vi "Procesare.vi"() -> ()   [LabVIEW 2024]
uses:
  <vilib>/vision/NI_Vision_Development_Module.lvlib
panel:
  out "Image":T1(plugin-control)
  out "Image 1D array":dbl[](array[numeric])
  out "Inputs":i32
  out "Dimensiune Imagine":i32[](array[numeric])
  out "Array":dbl[][](array[numeric])
  in  "Productivitate  minima":dbl
  in  "Ora  minima":dbl
  in  "Radiatie Solara minima":dbl
  in  "Viteza vant minima":dbl
  in  "Productivitate maxima":dbl
  in  "Ora maxima":dbl
  in  "Radiatie Solara maxima":dbl
  in  "Viteza Vant maxima":dbl
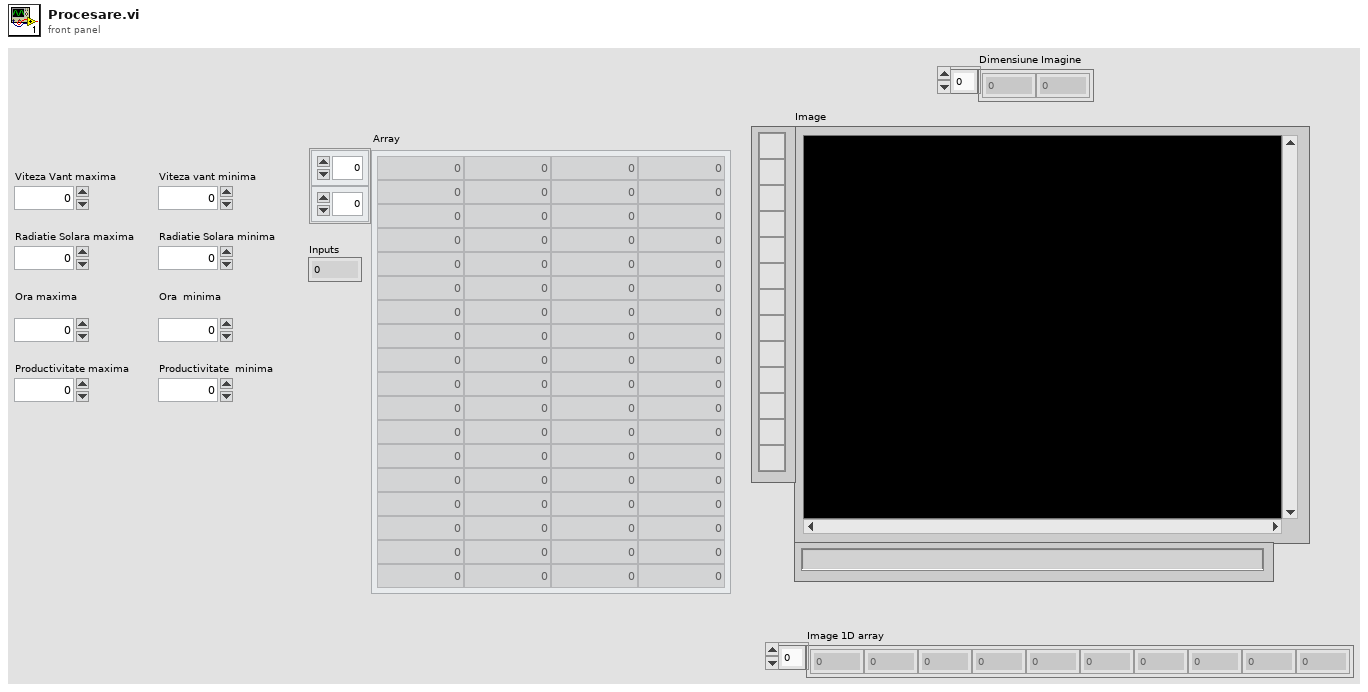
[diagram p1: front panel]
types:
  T1 = typedef "IMAQ Image.ctl" = refnum<image>
  T2 = typedef "Image Type" = u32
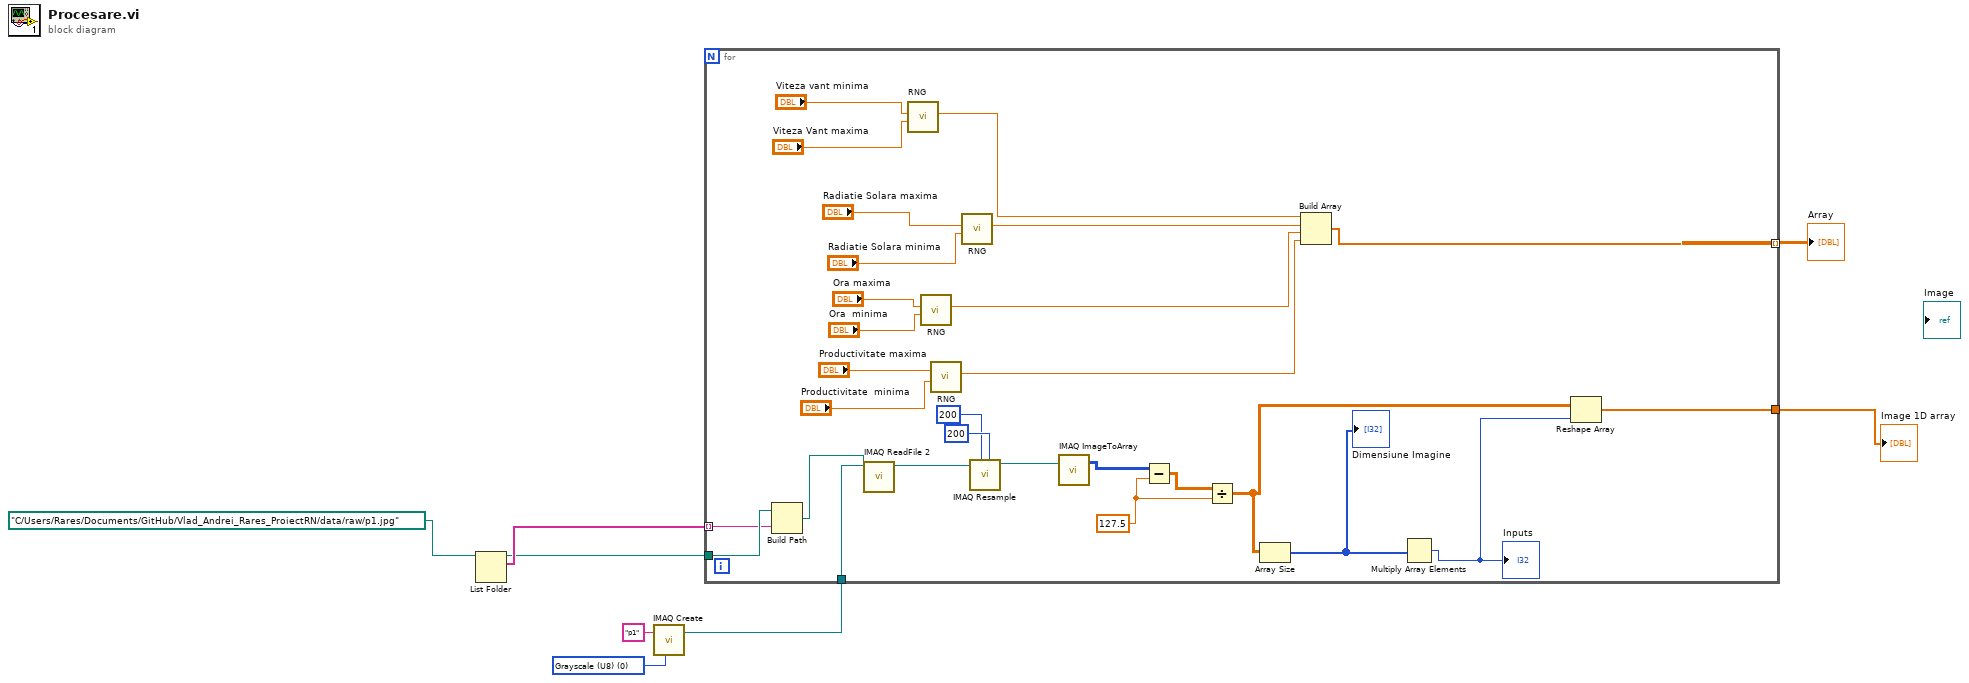
[diagram p0: block diagram]
diagram:
  w4 = T2 0 items=["Grayscale (U8)", "Grayscale (I16)", "Grayscale (SGL)", "Complex (CSG)", "RGB (U32)", "HSL (U32)", "RGB (U64)", "Grayscale (U16)"] ("Image Type")
  n1 = List Folder(path=path "C:/Users/Rares/Documents/GitHub/Vlad_Andrei_Rares_ProiectRN/data/raw/p1.jpg") -> (path out=w6:path, filenames=w7:string[])  [unwired: 3 in, 2 out]
  n2 = call "IMAQ Create"("Image Name"="p1", "Image Type"=w4) -> ("New Image"=w3:T1)  [unwired: 3 in, 1 out]
  n3 = for {
    tunnel: w7 -> [w35] mode=indexing
    tunnel: w6 -> [w36]
    tunnel: w3 -> [w34]
    tunnel: [w20] -> w2 mode=indexing
    tunnel: [w9] -> w1
    w13 = 127.5
    n4 = Build Path(base path=w36, name or relative path=w35) -> (appended path=w33:path)
    n5 = call "IMAQ ReadFile 2"("File Path"=w33, "Image"=w34) -> ("Image Out"=w17:T1)  [unwired: 5 in, 4 out]
    n6 = call "RNG.vi"("Minim"="Viteza Vant maxima", "Maxim"="Viteza vant minima") -> ("X val aleatoare"=w24:dbl)  [unwired: 9 in]
    n7 = call "RNG.vi"("Minim"="Ora  minima", "Maxim"="Ora maxima") -> ("X val aleatoare"=w22:dbl)  [unwired: 9 in]
    n8 = call "RNG.vi"("Minim"="Productivitate  minima", "Maxim"="Productivitate maxima") -> ("X val aleatoare"=w21:dbl)  [unwired: 9 in]
    n9 = call "RNG.vi"("Minim"="Radiatie Solara minima", "Maxim"="Radiatie Solara maxima") -> ("X val aleatoare"=w23:dbl)  [unwired: 9 in]
    n10 = call "IMAQ Resample"("X Resolution"=200, "Y Resolution"=200, "Image Src"=w17) -> ("Image Dst Out"=w16:T1)  [unwired: 7 in, 1 out]
    n11 = call "IMAQ ImageToArray"("Image"=w16) -> ("Image Pixels (I16)"=w15:i16[][])  [unwired: 3 in, 4 out]
    n12 = Subtract(x=w15, y=w13) -> (x-y=w14:dbl[][])
    n13 = Divide(x=w14, y=w13) -> (x/y=w10:dbl[][])
    n14 = Array Size(array=w10) -> (size(s)=w11:i32[])
    "Dimensiune Imagine" <- w11
    n15 = Build Array(w24, w23, w22, w21) -> (w20:dbl[])
    n16 = Multiply Array Elements(1:w11) -> (0:w12:i32)
    "Inputs" <- w12
    n17 = Reshape Array(w10, w12) -> (w9:dbl[])
  }
  "Array" <- w2
  "Image 1D array" <- w1
